vi "Status String.vi"(1 "Message":string) -> (0 "Status String":string)   [LabVIEW 2014]
panel:
  # "LICENSED MATERIALS – PROPERTY OF IBM\nCopyright IBM Corp. 2016,\nALL RIGHTS RESERVED"
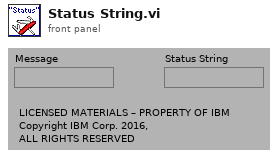
[diagram p1: front panel]
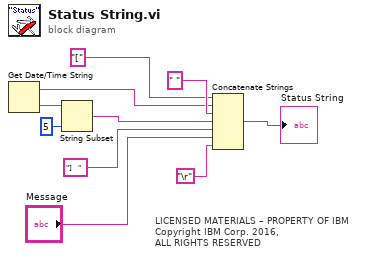
[diagram p0: block diagram]
diagram:
  # "LICENSED MATERIALS – PROPERTY OF IBM\nCopyright IBM Corp. 2016,\nALL RIGHTS RESERVED"
  n1 = Get Date/Time String() -> (date string=w7:string, time string=w1:string)  [unwired: 3 out]
  n2 = String Subset(string=w1, length (rest)=5 ("length (rest)")) -> (substring=w9:string)  [unwired: 1 out]
  n3 = Concatenate Strings("[" ("string"), w7, " " ("string"), w9, "]   " ("string"), "Message", "\r") -> (→"Status String":string)
